vi "LAKESHORE_12_01_2023_R_VS_T_DEMO_2.vi"() -> ()   [LabVIEW 2020]
panel:
  out "Resistance":dbl(graph)
  out "Temp":dbl(graph)
  out "Filename":string
  in  "Total iterations":i32
  out "Temperature":dbl
  in  "Average Number of readings \nper iterations":i32
  in  "Save data":bool
  out "Resistance(Ohms)":dbl
  in  "Channel":T1(ring)
  out "XY Graph":cluster{"X":dbl[], "Y":dbl[]}[](graph)
  in  "VISA resource name":refnum<visa-resource-name>
  # "LAKE SHORE 372"
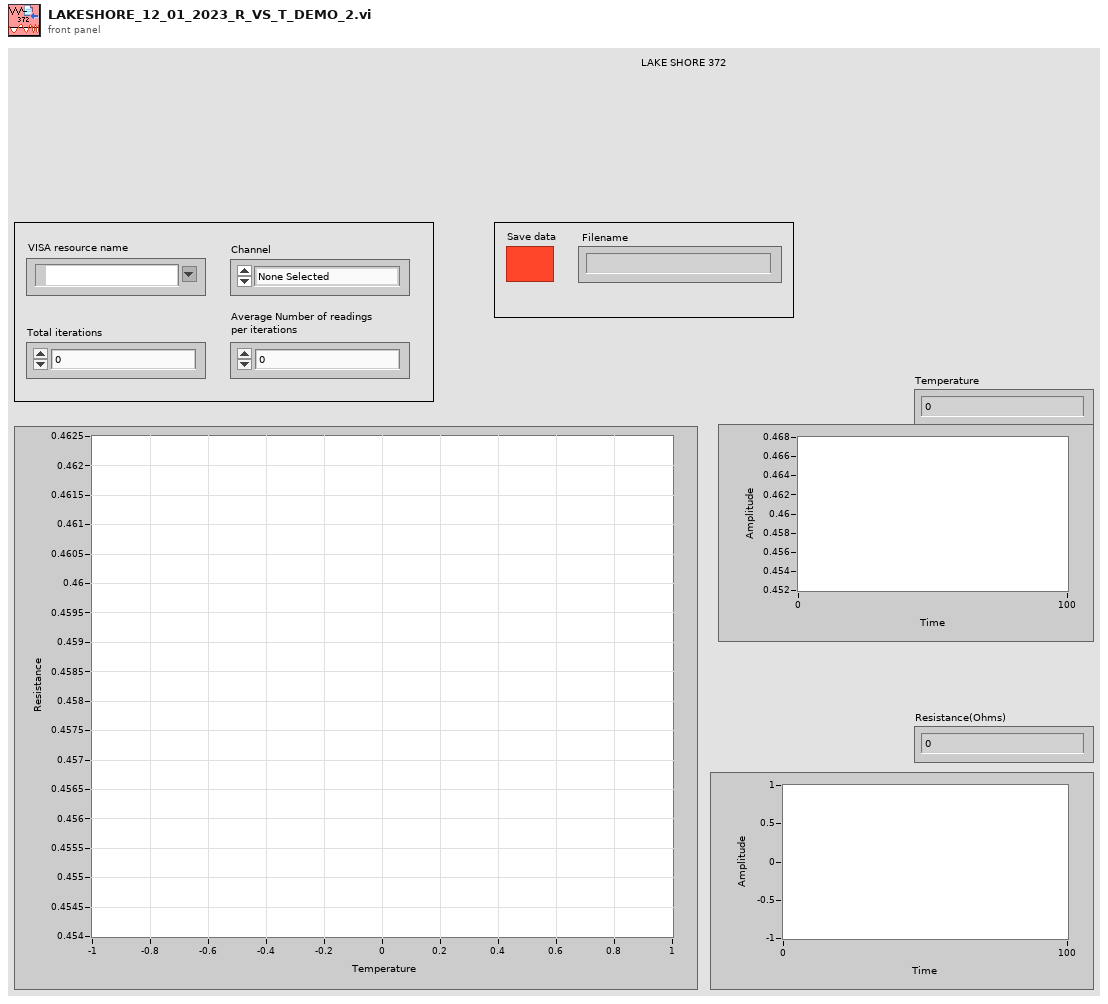
[diagram p1: front panel]
types:
  T1 = enum16{"None Selected", "1", "2", "3", "4", "5", "6", "7", "8", "9", "10", "11", "12", "13", "14", "15", "16"}
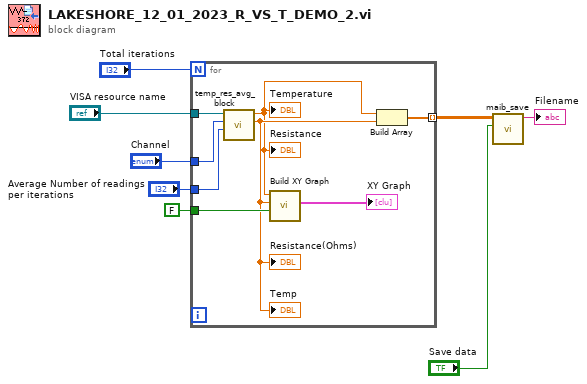
[diagram p0: block diagram]
diagram:
  n1 = for {
    N: "Total iterations" -> [_]
    tunnel: "VISA resource name" -> [w14]
    tunnel: FALSE ("Reset") -> [w15]
    tunnel: "Channel" -> [w13]
    tunnel: "Average Number of readings \nper iterations" -> [w12]
    tunnel: [w11] -> w3 mode=indexing
    n2 = call "temp_res_avg_block.vi"("Avg"=w12, "Channel in"=w13, "VISA Refnum in"=w14) -> ("Numeric"=w10:dbl, "Numeric 2"=w9:dbl)  [unwired: 7 in]
    "Resistance(Ohms)" <- w10
    "Temperature" <- w9
    "Temp" <- w10
    "Resistance" <- w9
    n3 = call "Build XY Graph"("Reset"=w15, "Y Input"=w10, "X Input"=w9) -> ("XY Graph"=→"XY Graph":cluster{"X":dbl[], "Y":dbl[]}[])  [unwired: 7 in, 1 out]
    n4 = Build Array(w9, w10) -> (w11:dbl[])
  }
  n5 = call "maib_save.vi"("Save data"="Save data", "Array"=w3) -> ("result string"=→"Filename":string)  [unwired: 9 in]
